vi "test_pre_filter_dll.vi"() -> ()   [LabVIEW 2016]
panel:
  out "Intensity Graph":dbl[][](graph)
  in  "Gaussian Filter Size":dbl=3.0
  in  "Mean Filter Size":i32=5
  out "Counter":i32
  out "Num Images":dbl=1000.0
  in  "AVI File for Simulated Raw B Scan Images":path=path "C:/Users/Applied Optics Group/Desktop/DCF Paper Data Processing/data/2020_08_04_2dcheckerboard_AF/Large_grid/OCT_raw_vol.avi"
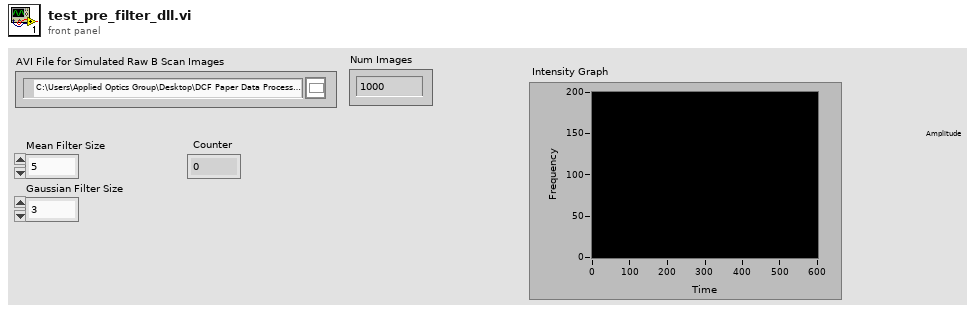
[diagram p1: front panel]
types:
  T1 = typedef "IMAQ Image.ctl" = refnum<image>
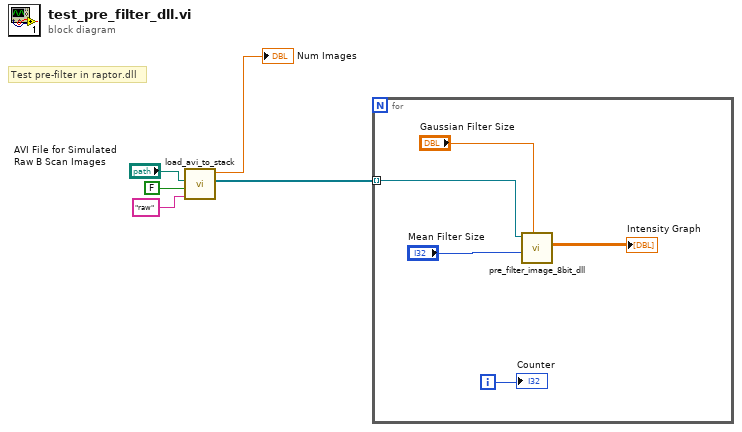
[diagram p0: block diagram]
diagram:
  # "Test pre-filter in raptor.dll"
  n1 = call "load_avi_to_stack.vi"("Image Prefix"="raw", "Preview"=FALSE, "AVI File"="AVI File for Simulated Raw B Scan Images") -> ("Image Array"=w1:T1[], "Num Images"=→"Num Images":dbl)  [unwired: 7 in]
  n2 = for {
    tunnel: w1 -> [w7] mode=indexing
    i -> [w10]
    n3 = call "pre_filter_image_8bit_dll.vi"("Gaussian Filter Size"="Gaussian Filter Size", "Mean Filter Size"="Mean Filter Size", "Input Image"=w7) -> ("Output Image Array"=→"Intensity Graph":dbl[][])  [unwired: 7 in, 1 out]
    "Counter" <- w10
  }
